vi "Plot Spectrum.vi"(8 "error in (no error)":errorcluster, 10 "Channel":u8, 11 "Micron Optics Recorder in":refnum<class "Spectrometer.lvclass">) -> (0 "error out":errorcluster, 3 "Micron Optics Recorder out":refnum<class "Spectrometer.lvclass">)   [LabVIEW 2016, in "Spectrometer.lvclass"]
uses:
  Spectrometer.lvclass
  C:/github/LabActor/Template Module/Template Module.lvclass
  Template Module/Template Module.lvclass/Template Module.ctl
  Spectrometer.lvclass/Spectrometer.ctl
  Template Module/Read Configuration.vi
  Read Spectrum Graph ref.vi
  NHMFL_Core/Libraries/Instruments/Spectrometer Driver/Spectrometer Driver.lvclass
  C:/github/NHMFL_Core/Libraries/Instruments/Instrument Driver/Instrument Driver.lvclass
  Read Spectrometer Driver.lvclass.vi
  NHMFL_Core/Libraries/Instruments/Instrument Driver/Write User configuration.vi
  Write Spectrometer Driver.lvclass.vi
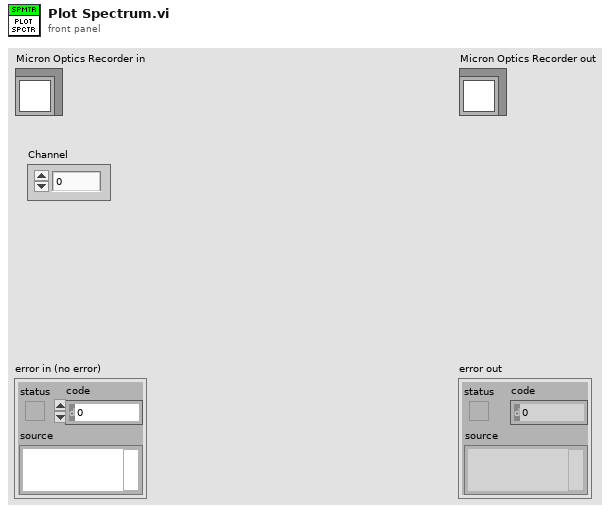
[diagram p1: front panel]
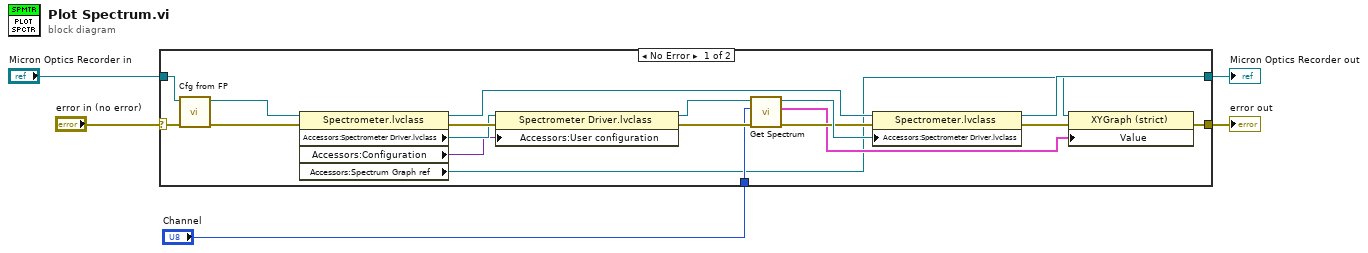
[diagram p0: block diagram]
diagram:
  n1 = case shown="No Error" "error in (no error)" {
    selector: "error in (no error)" -> [w14 w25]
    tunnel: [w17 w25] -> w4
    tunnel: [w21 w24] -> w2
    tunnel: "Micron Optics Recorder in" -> [w15 w24]
    tunnel: "Channel" -> [w7 _]
    frame No Error {
      n2 = call-dynamic "Cfg from FP.vi"("error in (no error)"=w14, "Measure Object in"=w15) -> ("error out"=w13:errorcluster, "Measure Object out"=w12:refnum<class "Spectrometer.lvclass">)  [unwired: 8 in]
      n3 = property class="Spectrometer.lvclass"(reference=w12, error in=w13) -> (reference out=w18:refnum<class "Spectrometer.lvclass">, error out=w23:errorcluster, "Accessors:Spectrometer Driver.lvclass"=w10:refnum<class "Spectrometer Driver.lvclass">, "Accessors:Configuration"=w8:variant, "Accessors:Spectrum Graph ref"=w6:refnum<vi>)
      n4 = property class="Spectrometer Driver.lvclass"(reference=w10, error in=w23, "Accessors:User configuration"=w8) -> (reference out=w9:refnum<class "Spectrometer Driver.lvclass">, error out=w11:errorcluster)
      n5 = call-dynamic "Get Spectrum.vi"("error in (no error)"=w11, "Channel"=w7, "Spectrometer Driver in"=w9) -> ("error out"=w19:errorcluster, "Spectrum Graph"=w16:cluster{dbl[], "Spectrum, db":dbl[]}[], "Spectrometer Driver out"=w20:refnum<class "Spectrometer Driver.lvclass">)  [unwired: 6 in]
      n6 = property class="Spectrometer.lvclass"(reference=w18, error in=w19, "Accessors:Spectrometer Driver.lvclass"=w20) -> (reference out=w21:refnum<class "Spectrometer.lvclass">, error out=w22:errorcluster)
      n7 = property class="XYGraph (strict)"(reference=w6, error in=w22, "Value"=w16) -> (error out=w17:errorcluster)  [unwired: 1 out]
    }
    frame Error {
    }
  }
  "error out" <- w4
  "Micron Optics Recorder out" <- w2
